vi "Find Nested Projects.vi"(8 "error in (no error)":errorcluster, 11 "Projext Path":path) -> (0 "error out":errorcluster, 3 "Array":path[](array[path]))   [LabVIEW 2020, in "Test Finder.lvclass"]
uses:
  Test Finder.lvclass
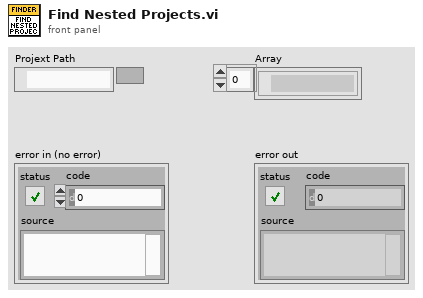
[diagram p1: front panel]
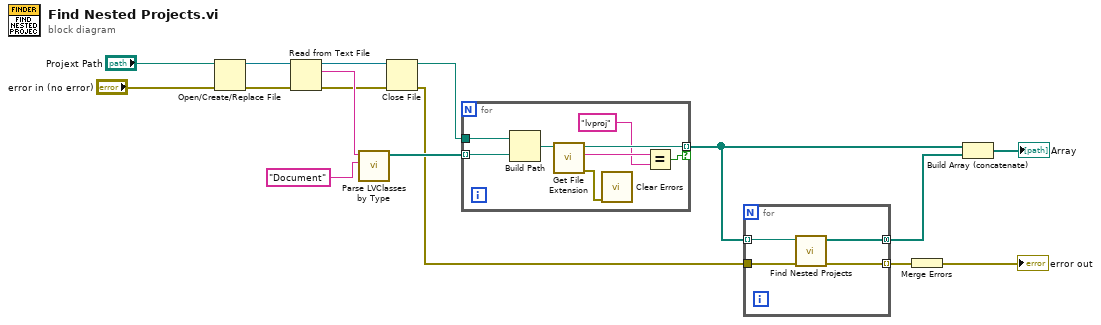
[diagram p0: block diagram]
diagram:
  n1 = Open/Create/Replace File(file path (use dialog)="Projext Path", error in="error in (no error)") -> (refnum out=w9:refnum<file>, error out=w10:errorcluster)  [unwired: 4 in, 1 out]
  n2 = Read from Text File(file (use dialog)=w9, error in=w10) -> (refnum out=w11:refnum<file>, text=w14:string, error out=w12:errorcluster)  [unwired: 2 in, 1 out]
  n3 = call "Parse LVClasses by Type.vi"("Type"="Document", "Input"=w14) -> ("Relative Paths"=w7:path[])  [unwired: 9 in]
  n4 = Close File(refnum=w11, error in=w12) -> (path=w15:path, error out=w3:errorcluster)
  n5 = for {
    tunnel: w15 -> [w24]
    tunnel: w7 -> [w23] mode=indexing
    tunnel: [w21] -> w6 mode=indexing if=w17
    n6 = Build Path(base path=w24, name or relative path=w23) -> (appended path=w22:path)
    n7 = call <vilib>:"Get File Extension.vi"("file"=w22) -> ("error out"=w18:errorcluster, "lowercase file extension"=w20:string, "dup file"=w21:path)  [unwired: 6 in, 2 out]
    n8 = call <vilib>:"Clear Errors.vi"("error in (no error)"=w18) -> ()  [unwired: 5 in, 2 out]
    n9 = Equal?(x=w20, y="lvproj") -> (x = y?=w17:bool)
  }
  n10 = for {
    tunnel: w6 -> [w28] mode=indexing
    tunnel: [w27] -> w4 mode=concatenating
    tunnel: w3 -> [w26]
    tunnel: [w25] -> w2 mode=indexing
    n11 = call "Find Nested Projects.vi"("error in (no error)"=w26, "Projext Path"=w28) -> ("error out"=w25:errorcluster, "Array"=w27:path[])  [unwired: 8 in]
  }
  n12 = Merge Errors(w2) -> (→"error out":errorcluster)
  n13 = Build Array (concatenate)(w6, w4) -> (→"Array":path[])
